vi "GlobalVariableDemo.vi"() -> ()   [LabVIEW 2019]
uses:
  LightsOnGlobal.vi
panel:
  out "Light 2":bool
  out "Light 1":bool
  in  "Boolean":bool
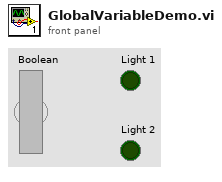
[diagram p1: front panel]
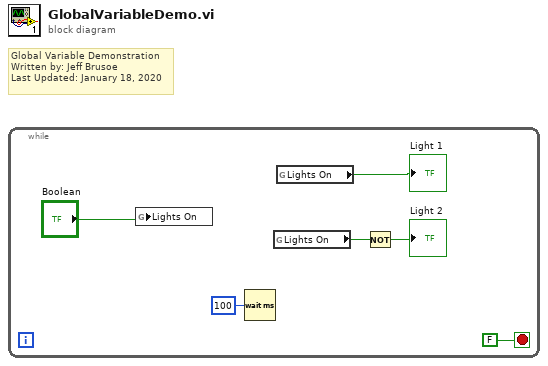
[diagram p0: block diagram]
diagram:
  # "Global Variable Demonstration\nWritten by: Jeff Brusoe\nLast Updated: January 18, 2020"
  n1 = while {
    stop <- FALSE stop-if-true
    n2 = global write "LightsOnGlobal.vi" "Lights On"("Boolean") -> ()
    n3 = Wait (ms)(milliseconds to wait=u32 100) -> ()  [unwired: 1 out]
    n4 = global read "LightsOnGlobal.vi" "Lights On"() -> (w3:bool)
    n5 = global read "LightsOnGlobal.vi" "Lights On"() -> (→"Light 1":bool)
    n6 = Not(x=w3) -> (.not. x?=→"Light 2":bool)
  }
